vi "MatchPos2RECTwAngle (SubVI).vi"(11 "Match element":T1) -> (3 "Rectangle with Angle":cluster{"x":sgl, "y":sgl, dbl, dbl, "Angle":sgl})   [LabVIEW 2016]
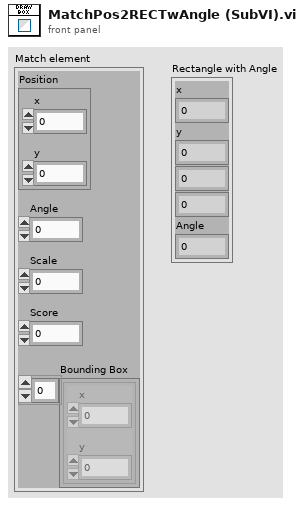
[diagram p1: front panel]
types:
  T1 = cluster{"Position":cluster{"x":sgl, "y":sgl}, "Angle":sgl, "Scale":sgl, "Score":sgl, "Bounding Box":cluster{"x":sgl, "y":sgl}[]}
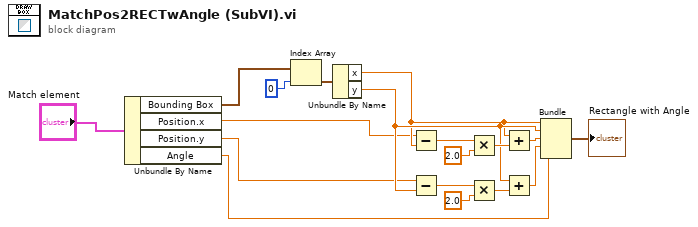
[diagram p0: block diagram]
diagram:
  n1 = Unbundle By Name("Match element") -> ("Bounding Box"=w5:cluster{"x":sgl, "y":sgl}[], "Position.x"=w4:sgl, "Position.y"=w3:sgl, "Angle"=w2:sgl)
  n2 = Index Array(array=w5, index=0) -> (element=w8:cluster{"x":sgl, "y":sgl})
  n3 = Unbundle By Name(w8) -> ("x"=w11:sgl, "y"=w12:sgl)
  n4 = Subtract(x=w4, y=w11) -> (x-y=w15:sgl)
  n5 = Subtract(x=w3, y=w12) -> (x-y=w17:sgl)
  n6 = Multiply(x=w15, y=2.0) -> (x*y=w16:dbl)
  n7 = Multiply(x=w17, y=2.0) -> (x*y=w18:dbl)
  n8 = Add(x=w11, y=w16) -> (x+y=w9:dbl)
  n9 = Add(x=w12, y=w18) -> (x+y=w10:dbl)
  n10 = Bundle("x"=w11, "y"=w12, w9, w10, "Angle"=w2) -> (→"Rectangle with Angle":cluster{"x":sgl, "y":sgl, dbl, dbl, "Angle":sgl})  [unwired: 1 in]
